vi "Kaelus PIM Load Test Sets in Tree.vi"(7 "Base Configuration":T1={"host IP (localhost)"="", "host Port"=0, "Model"="", "Serial Number(s)"="", "Calibration Date"=3388.0, "Dual Port?"=FALSE, "DeviceNames"=[], "Parameters"={"TX1start"=0.0, "TX1stop"=0.0, "TX1pmax"=0.0, "TX2start"=0.0, "TX2stop"=0.0, "TX2pmax"=0.0, "RXstart"=0.0, "RXstop"=0.0}, "Interface"=enum."PIM Web Engine"} {"Calibration Date" format="%.2f"; "Parameters"."TX2pmax" format="%.1f"; "Parameters"."TX1pmax" format="%.1f"; "Parameters"."RXstop" format="%.1f"; "Parameters"."RXstart" format="%.1f"; "Parameters"."TX2stop" format="%.1f"; "Parameters"."TX2start" format="%.1f"; "Parameters"."TX1stop" format="%.1f"; "Parameters"."TX1start" format="%.1f"}, 8 "error in (no error)":errorcluster, 10 "TestSet Definitions":T3[](array[typedef]), 11 "Tree Control Reference":refnum<vi>) -> (0 "error out":errorcluster, 2 "Populated Configurations":T1[](array[typedef]) {"Calibration Date" format="%.2f"; "Parameters"."TX2pmax" format="%.1f"; "Parameters"."TX1pmax" format="%.1f"; "Parameters"."RXstop" format="%.1f"; "Parameters"."RXstart" format="%.1f"; "Parameters"."TX2stop" format="%.1f"; "Parameters"."TX2start" format="%.1f"; "Parameters"."TX1stop" format="%.1f"; "Parameters"."TX1start" format="%.1f"})   [LabVIEW 2011]
uses:
  PIM Configuration.ctl
  PIM Interface Language.ctl
  BPIMCore EXT/HW IO/Test Set Definition.ctl
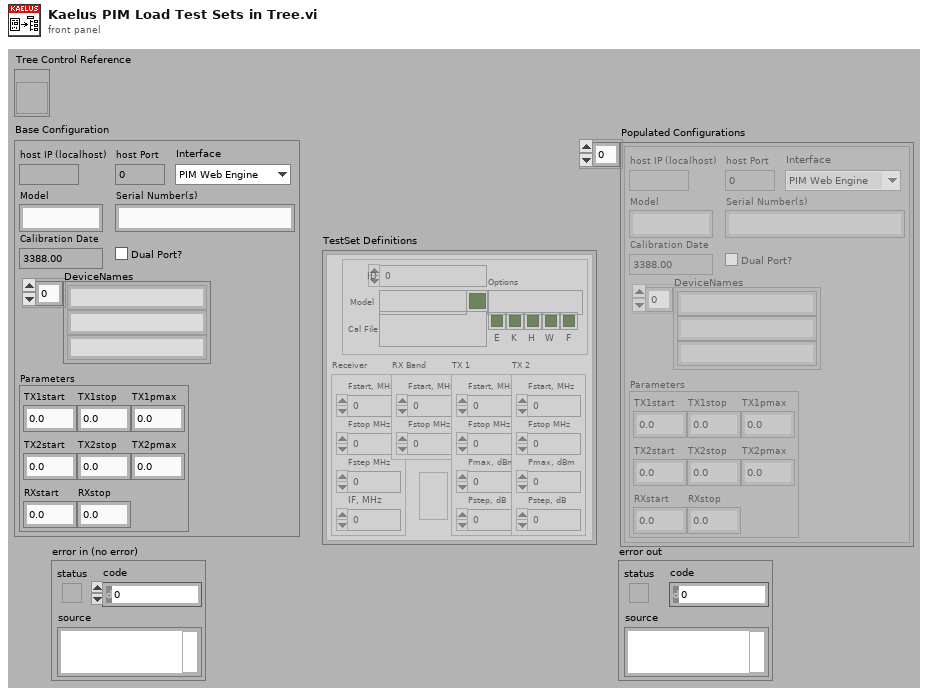
[diagram p1: front panel]
types:
  T1 = typedef "PIM Configuration.ctl" = cluster{"host IP (localhost)":string, "host Port":u16, "Model":string, "Serial Number(s)":string, "Calibration Date":dbl, "Dual Port?":bool, "DeviceNames":string[], "Parameters":cluster{"TX1start":dbl, "TX1stop":dbl, "TX1pmax":dbl, "TX2start":dbl, "TX2stop":dbl, "TX2pmax":dbl, "RXstart":dbl, "RXstop":dbl}, "Interface":T2}
  T2 = typedef "PIM Interface Language.ctl" = enum16{"PIM Web Engine", "PIM HW Engine"}
  T3 = typedef "Test Set Definition.ctl" = cluster{"General":cluster{"ID":u32, "Model":string, "Dual Port?":bool, "Options":string, "Options":cluster{"E":bool, "K":bool, "H":bool, "W":bool, "F":bool}, "Cal File":path}, "Receiver":cluster{"Fstart, MHz":dbl, "Fstop MHz":dbl, "Fstep MHz":dbl, "IF, MHz":dbl}, "RX Band":cluster{"Fstart, MHz":dbl, "Fstop MHz":dbl}, "TX 1":cluster{"Fstart, MHz":dbl, "Fstop MHz":dbl, "Pmax, dBm":dbl, "Pstep, dB":dbl}, "TX 2":cluster{"Fstart, MHz":dbl, "Fstop MHz":dbl, "Pmax, dBm":dbl, "Pstep, dB":dbl}, "Low-side?":bool}
  T4 = cluster{"version":u8, "date":string, "serial number":string, "datestamp":dbl, "validCal?":bool}
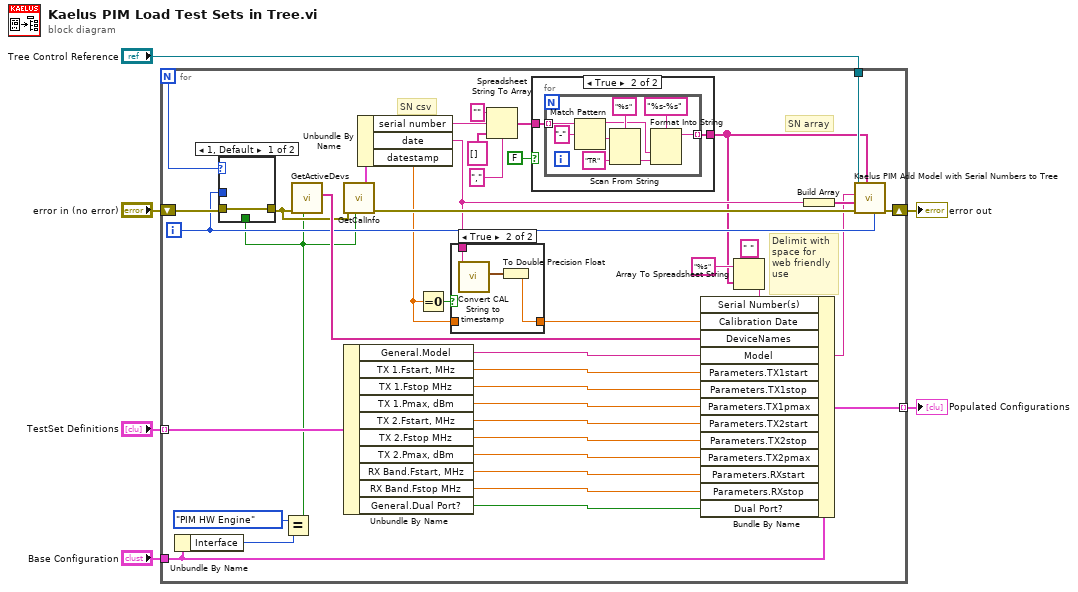
[diagram p0: block diagram]
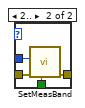
[diagram p4: hidden frame]
diagram:
  n1 = for {
    N -> [w44]
    shift-right: [w34] -> w3
    shift-left: "error in (no error)" -> [w45]
    tunnel: "TestSet Definitions" -> [w42] mode=indexing
    tunnel: "Base Configuration" -> [w20]
    tunnel: "Tree Control Reference" -> [w32]
    tunnel: [w31] -> w2 mode=indexing
    i -> [w30]
    # "Delimit with\nspace for \nweb friendly\nuse"
    # "SN csv"
    # "SN array"
    n2 = Unbundle By Name(w20) -> ("Interface"=w19:T2)
    n3 = Equal?(x=PIM_Interface_Language."PIM HW Engine" ("Interface"), y=w19) -> (x = y?=w18:bool)
    n4 = case shown="1, Default" w44 {
      tunnel: w30 -> [_ w67]
      tunnel: w45 -> [w63 w66]
      tunnel: [w63 w65] -> w21
      tunnel: w18 -> [_ w64]
      frame 1, Default {
      }
      frame 2.. {
        n5 = call "SetMeasBand.vi"("Legacy (f)?"=w64, "error in (no error)"=w66, "Band Index"=w67) -> ("error out"=w65:errorcluster)  [unwired: 8 out]
      }
    }
    n6 = call "GetActiveDevs.vi"("Legacy (f)?"=w18, "error in (no error)"=w21) -> ("Active Device Names"=w43:string[])  [unwired: 8 in, 1 out]
    n7 = call "GetCalInfo.vi"("Legacy (f)?"=w18, "error in (no error)"=w21) -> ("error out"=w35:errorcluster, "CalInfo"=w46:T4)  [unwired: 8 out]
    n8 = Unbundle By Name(w42) -> ("General.Model"=w29:string, "TX 1.Fstart, MHz"=w41:dbl, "TX 1.Fstop MHz"=w40:dbl, "TX 1.Pmax, dBm"=w27:dbl, "TX 2.Fstart, MHz"=w39:dbl, "TX 2.Fstop MHz"=w38:dbl, "TX 2.Pmax, dBm"=w26:dbl, "RX Band.Fstart, MHz"=w37:dbl, "RX Band.Fstop MHz"=w36:dbl, "General.Dual Port?"=w25:bool)
    n9 = Unbundle By Name(w46) -> ("serial number"=w13:string, "date"=w28:string, "datestamp"=w9:dbl)
    n10 = Equal To 0?(x=w9) -> (x = 0?=w10:bool)
    n11 = case shown="True" w10 {
      tunnel: w28 -> [_ w61]
      tunnel: w9 -> [w59 _]
      tunnel: [w59 w60] -> w8
      frame False {
      }
      frame True {
        n12 = call "Convert CAL String to timestamp.vi"("abbreviated date string"=w61) -> ("time stamp"=w62:timestamp)  [unwired: 10 out]
        n13 = To Double Precision Float(number=w62) -> (double precision float=w60:dbl)
      }
    }
    n14 = Spreadsheet String To Array(delimiter (Tab)=",", format string="", spreadsheet string=w13, array type (2D Dbl)=string[] []) -> (array=w16:string[])
    n15 = case shown="True" FALSE {
      tunnel: w16 -> [w47 w49]
      tunnel: [w47 w48] -> w12
      frame False {
      }
      frame True {
        n16 = for {
          tunnel: w49 -> [w57] mode=indexing
          tunnel: [w50] -> w48 mode=indexing
          n17 = Match Pattern(string=w57, regular expression="-") -> (before substring=w51:string, after substring=w54:string)  [unwired: 1 in, 2 out]
          n18 = Scan From String(format string="%s", input string=w54, default 1="TR" ("format string")) -> (output 1=w52:string)  [unwired: 2 in, 3 out]
          n19 = Format Into String(format string="%s-%s", w51, w52) -> (resulting string=w50:string)  [unwired: 2 in, 1 out]
        }
      }
    }
    n20 = Array To Spreadsheet String(delimiter (Tab)=" ", array=w12, 3:"%s" ("format string")) -> (spreadsheet string=w24:string)
    n21 = Bundle By Name(cluster=w20, "Serial Number(s)"=w24, "Calibration Date"=w8, "DeviceNames"=w43, "Model"=w29, "Parameters.TX1start"=w41, "Parameters.TX1stop"=w40, "Parameters.TX1pmax"=w27, "Parameters.TX2start"=w39, "Parameters.TX2stop"=w38, "Parameters.TX2pmax"=w26, "Parameters.RXstart"=w37, "Parameters.RXstop"=w36, "Dual Port?"=w25) -> (w31:T1)
    n22 = Build Array(w28) -> (w33:string[])
    n23 = call "Kaelus PIM Add Model with Serial Numbers to Tree.vi"("Instrument Index"=w30, "Model Serial Numbers"=w12, "error in (no error)"=w35, "Model Descriptive Columns"=w33, "Model Name"=w29, "Tree Control Reference"=w32) -> ("error out"=w34:errorcluster)  [unwired: 5 in]
  }
  "error out" <- w3
  "Populated Configurations" <- w2
